vi "Pull File.vi"(6 "Type (Binary)":u16(ring)=1 items=["ASCII", "Binary"], 8 "error in (no error)":errorcluster, 9 "Local FilePath":path, 10 "FileName":string, 11 "FTP in":refnum<class "FTP.lvclass">) -> (0 "error out":errorcluster, 3 "FTP out":refnum<class "FTP.lvclass">)   [LabVIEW 2013, in "FTP.lvlib" / "FTP.lvclass"]
doc: "This vi will \"pull\" a file from the remote ftp server to a location on the local directory. The file will be pulled from the current directory on the ftp server. Use the \"Change Directory.vi\" to change the current remote directory. The user is allowed to select the type of file to transfer. The default is a binary file, which is the preferred method of transferring files."
uses:
  FTP.lvclass
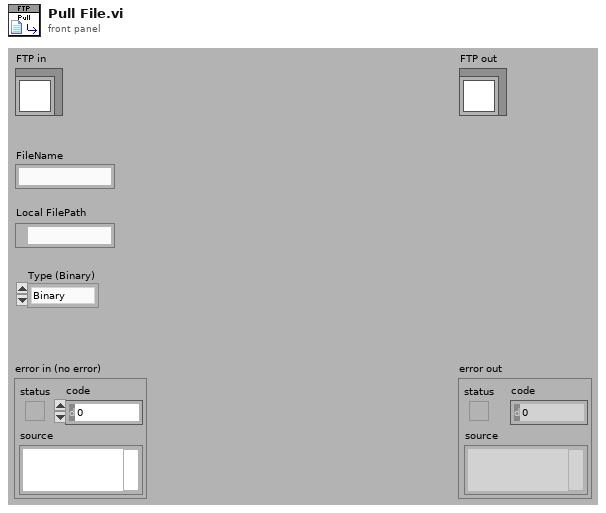
[diagram p1: front panel]
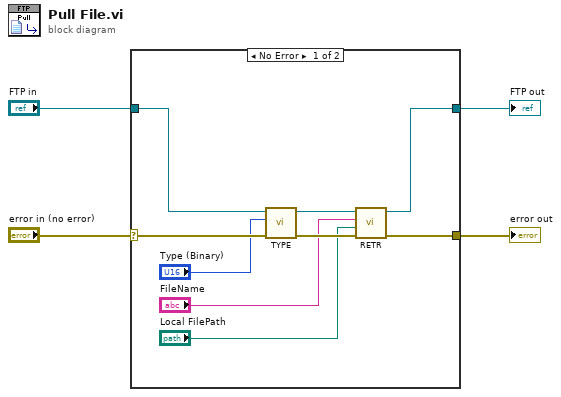
[diagram p0: block diagram]
diagram:
  n1 = case shown="No Error" "error in (no error)" {
    selector: "error in (no error)" -> [w12 w15]
    tunnel: [w8 w15] -> w3
    tunnel: [w9 w14] -> w1
    tunnel: "FTP in" -> [w13 w14]
    frame No Error {
      n2 = call "TYPE.vi"("error in (no error)"=w12, "Type"="Type (Binary)", "FTP in"=w13) -> ("error out"=w10:errorcluster, "FTP out"=w11:refnum<class "FTP.lvclass">)  [unwired: 7 in]
      n3 = call "RETR.vi"("error in (no error)"=w10, "Local FilePath"="Local FilePath", "FileName"="FileName", "FTP in"=w11) -> ("error out"=w8:errorcluster, "FTP out"=w9:refnum<class "FTP.lvclass">)  [unwired: 6 in]
    }
    frame Error {
    }
  }
  "error out" <- w3
  "FTP out" <- w1
